vi "Model Initial Values - Get Model Info.vi"(8 "error in (no error)":errorcluster, 11 "ID in":T2 format="%.0x") -> (0 "error out":errorcluster, 2 "output cluster":T1, 3 "ID out":T2 format="%.0x")   [LabVIEW 2015, in "Model Initial Values Custom Device.lvlib"]
uses:
  Model Initial Values Custom Device.lvlib
  <vilib>/NI Veristand/Custom Device API/Custom Device Item Ref.ctl
  NationalInstruments.VeriStand.SystemDefinitionAPI
  <vilib>/NI Veristand/Custom Device Offline API/Custom Device Offline API.lvlib
  <vilib>/NI Veristand/Custom Device API/Custom Device API.lvlib
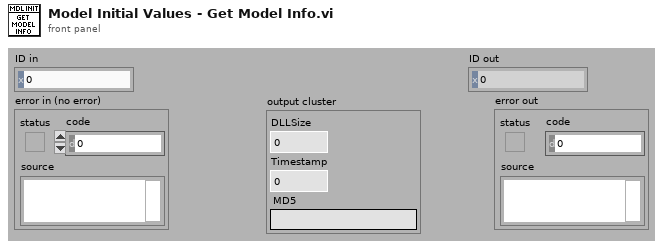
[diagram p1: front panel]
types:
  T1 = cluster{"DLLSize":i32, "Timestamp":dbl, "MD5":string}
  T2 = typedef "Custom Device API.lvlib/Custom Device Item Ref.ctl" = u64
  T3 = cluster{"DLLSize":i32, "ModelTimestamp":dbl, "MD5":string}
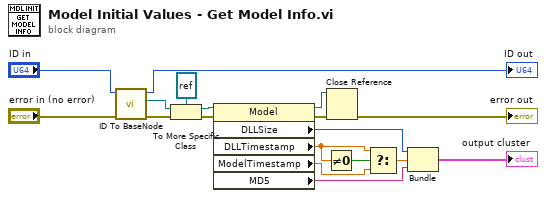
[diagram p0: block diagram]
diagram:
  n1 = call <vilib>:"ID To BaseNode.vi"("error in (no error)"="error in (no error)", "ID in"="ID in") -> ("error out"=w16:errorcluster, "BaseNode"=w18:refnum<k24>, "ID out"=→"ID out":u64)  [unwired: 7 in]
  n2 = To More Specific Class(target class=refnum<k24> refnum ("BaseNodeType"), reference=w18, error in=w16) -> (specific class reference=w15:refnum<k24>, error out=w14:errorcluster)
  n3 = property class="Model"(reference=w15, error in=w14) -> (reference out=w8:refnum<k24>, error out=w7:errorcluster, "DLLSize"=w13:i32, "DLLTimestamp"=w4:dbl, "ModelTimestamp"=w5:dbl, "MD5"=w2:string)
  n4 = Not Equal To 0?(x=w4) -> (x != 0?=w6:bool)
  n5 = Close Reference(reference=w8, error in (no error)=w7) -> (error out=→"error out":errorcluster)
  n6 = Select(t=w4, s=w6, f=w5) -> (s? t:f=w3:dbl)
  n7 = Bundle("DLLSize"=w13, "ModelTimestamp"=w3, "MD5"=w2) -> (→"output cluster":T3)  [unwired: 1 in]
